vi "switch.vi"(1 "error in (no error)":errorcluster, 2 "vi close":refnum<vi>, 3 "vi open":refnum<vi>) -> (0 "error out":errorcluster)   [LabVIEW 2013]
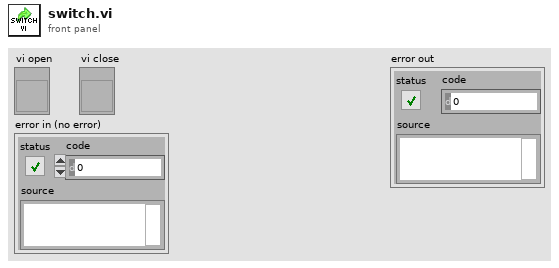
[diagram p1: front panel]
types:
  T1 = enum32{"Bad", "Idle", "Run top level", "Running"}
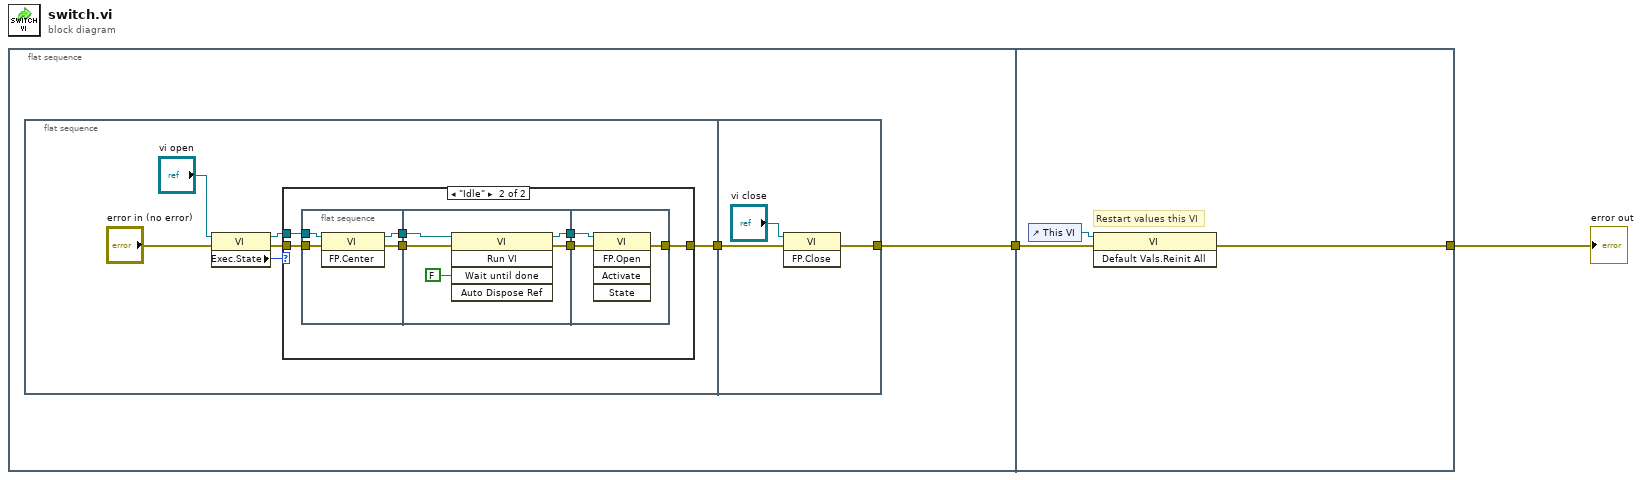
[diagram p0: block diagram]
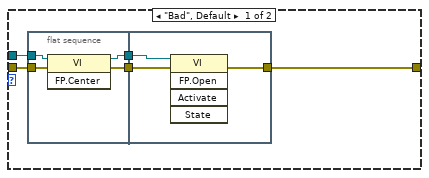
[diagram p2: hidden frame]
diagram:
  n1 = flat-sequence {
    tunnel: [w4] -> w1
    tunnel: [w46] -> w2
    tunnel: w1 -> [w45]
    frame #0 {
      n2 = flat-sequence {
        tunnel: [w5] -> w3
        tunnel: [w43] -> w4
        tunnel: w3 -> [w42]
        frame #0 {
          n3 = property class="VI"(reference="vi open", error in="error in (no error)") -> (reference out=w8:refnum<vi>, error out=w7:errorcluster, "Exec.State"=w9:T1)
          n4 = case shown="\"Idle\"" w9 {
            tunnel: w8 -> [w15 w29]
            tunnel: w7 -> [w14 w26]
            tunnel: [w11 w23] -> w5
            frame "Bad", Default {
              n5 = flat-sequence {
                tunnel: w15 -> [w19]
                tunnel: w14 -> [w18]
                tunnel: [w17] -> w13
                tunnel: [w16] -> w12
                tunnel: w13 -> [w22]
                tunnel: w12 -> [w21]
                tunnel: [w20] -> w11
                frame #0 {
                  n6 = invoke class="VI" method="FP.Center"(reference=w19, error in=w18) -> (reference out=w16:refnum<vi>, error out=w17:errorcluster)  [unwired: 1 in, 1 out]
                }
                frame #1 {
                  n7 = invoke class="VI" method="FP.Open"(reference=w21, error in=w22) -> (error out=w20:errorcluster)  [unwired: 3 in, 4 out]
                }
              }
            }
            frame "Idle" {
              n8 = flat-sequence {
                tunnel: w29 -> [w33]
                tunnel: [w32] -> w27
                tunnel: w26 -> [w31]
                tunnel: [w30] -> w25
                tunnel: [w37] -> w28
                tunnel: w27 -> [w36]
                tunnel: w25 -> [w35]
                tunnel: [w34] -> w24
                tunnel: w28 -> [w41]
                tunnel: w24 -> [w40]
                tunnel: [w39] -> w23
                frame #0 {
                  n9 = invoke class="VI" method="FP.Center"(reference=w33, error in=w31) -> (reference out=w32:refnum<vi>, error out=w30:errorcluster)  [unwired: 1 in, 1 out]
                }
                frame #1 {
                  n10 = invoke class="VI" method="Run VI"(reference=w36, error in=w35, "Wait until done"=FALSE ("Wait Until Done")) -> (reference out=w37:refnum<vi>, error out=w34:errorcluster)  [unwired: 2 in, 3 out]
                }
                frame #2 {
                  n11 = invoke class="VI" method="FP.Open"(reference=w41, error in=w40) -> (error out=w39:errorcluster)  [unwired: 3 in, 4 out]
                }
              }
            }
          }
        }
        frame #1 {
          n12 = invoke class="VI" method="FP.Close"(reference="vi close", error in=w42) -> (error out=w43:errorcluster)  [unwired: 1 in, 2 out]
        }
      }
    }
    frame #1 {
      # "Restart values this VI"
      n13 = control-ref of="This VI"() -> (w47:refnum<vi>)
      n14 = invoke class="VI" method="Default Vals.Reinit All"(reference=w47, error in=w45) -> (error out=w46:errorcluster)  [unwired: 1 in, 2 out]
    }
  }
  "error out" <- w2
